vi "File.Files and SubFolders.vi"(8 "error in":errorcluster, 9 "Dest Path":path, 10 "Folder":path, 11 "Zip File":i64) -> (0 "error out":errorcluster, 2 "Dest Path Out":path, 3 "Zip File Out":i64)   [LabVIEW 2024]
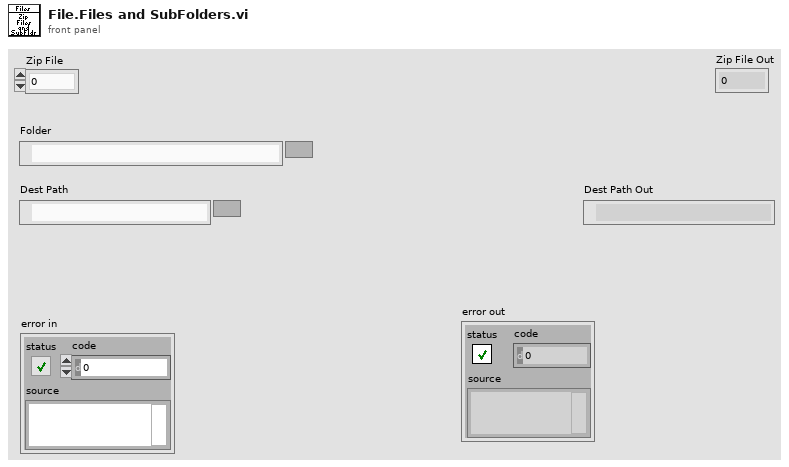
[diagram p1: front panel]
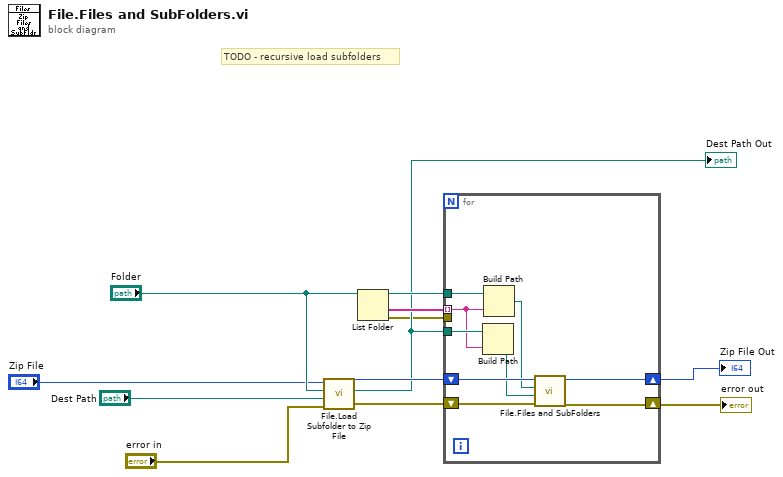
[diagram p0: block diagram]
diagram:
  # "TODO - recursive load subfolders"
  n1 = call "File.Load Subfolder to Zip File.vi"("error in"="error in", "Dest Path"="Dest Path", "Source Folder"="Folder", "Zip File"="Zip File") -> ("error out"=w8:errorcluster, "Dest Path Out"=w2:path, "Zip File Out"=w9:i64)  [unwired: 5 in]
  "Dest Path Out" <- w2
  n2 = List Folder(path="Folder") -> (path out=w10:path, folder names=w11:string[], error out=w1:errorcluster)  [unwired: 3 in, 1 out]
  n3 = for {
    tunnel: w11 -> [w14] mode=indexing
    tunnel: w10 -> [w17]
    shift-right: [w20] -> w3
    shift-left: w9 -> [w21]
    shift-right: [w19] -> w6
    shift-left: w8 -> [w18]
    tunnel: w2 -> [w15]
    tunnel: w1 -> [_]
    n4 = Build Path(base path=w15, name or relative path=w14) -> (appended path=w13:path)
    n5 = Build Path(base path=w17, name or relative path=w14) -> (appended path=w16:path)
    n6 = call "File.Files and SubFolders.vi"("error in"=w18, "Dest Path"=w13, "Folder"=w16, "Zip File"=w21) -> ("error out"=w19:errorcluster, "Zip File Out"=w20:i64)  [unwired: 5 in, 1 out]
  }
  "error out" <- w6
  "Zip File Out" <- w3
